vi "Initialize.vi"(8 "error in":errorcluster, 9 "Number of Channels":u32=1, 10 "Plugin Name":string, 11 "Power Control in":refnum<class "Power Control.lvclass">) -> (0 "error out":errorcluster, 3 "Power Control out":refnum<class "Power Control.lvclass">)   [LabVIEW 2023, in "Power Control.lvclass"]
uses:
  Power Control.lvclass
  Power Control.lvclass/Power Control.ctl
  <vilib>/ADAS Replay HIL/Channels/Tag Wrapper/Polymorphic/Open Consumer Tag (Double).vi
  <vilib>/ADAS Replay HIL/Channels/Tag Wrapper/Polymorphic/Open Consumer Tag (Double).vi/bacb721e-673a-491a-accd-959f2e1f334e.vi
  <vilib>/ADAS Replay HIL/Channels/Tag Wrapper/Polymorphic/Open Consumer Tag (Double).vi/bacb721e-673a-491a-accd-959f2e1f334e.vi/c28b0ead-42ad-4072-80a2-aca7f2bd7ce3.vi
  <vilib>/ADAS Replay HIL/AdasHilServices/AdasHilServices Fill In Error Info Ex.vi
  <vilib>/ADAS Replay HIL/Channels/Tag Wrapper/Tag Wrapper.lvlib
  Utilities.lvlib
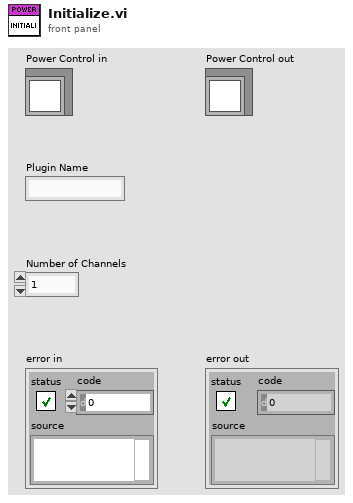
[diagram p1: front panel]
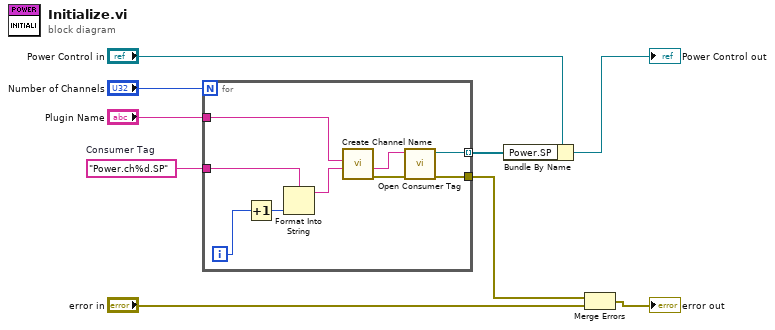
[diagram p0: block diagram]
diagram:
  w8 = "Power.ch%d.SP"  # Consumer Tag
  n1 = for {
    N: "Number of Channels" -> [_]
    tunnel: w8 -> [w12]
    tunnel: [w16] -> w7
    tunnel: "Plugin Name" -> [w15]
    tunnel: [w14] -> w2 mode=indexing
    i -> [w11]
    n2 = Increment(x=w11) -> (x+1=w10:i32)
    n3 = Format Into String(format string=w12, w10) -> (resulting string=w13:string)  [unwired: 2 in, 1 out]
    n4 = call "Create Channel Name.vi"("Channel Name"=w13, "Plugin Name"=w15) -> ("error out"=w17:errorcluster, "Data Channel Name"=w18:string)  [unwired: 8 in]
    n5 = call-poly <vilib>:"Open Consumer Tag.vi"("error in"=w17, "Channel Name"=w18) -> ("error out"=w16:errorcluster, "ADAS HIL Channel"=w14:refnum<k21>)  [unwired: 8 in]
  }
  n6 = Bundle By Name(cluster="Power Control in", "Power.SP"=w2) -> (→"Power Control out":refnum<class "Power Control.lvclass">)
  n7 = Merge Errors(w7, "error in") -> (→"error out":errorcluster)
